vi "myRIO_BRig_RT_dataExp_laser1_Power_max.vi"() -> (2 "output_laser1_Power_max":i32)   [LabVIEW 2014]
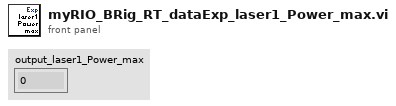
[diagram p1: front panel]
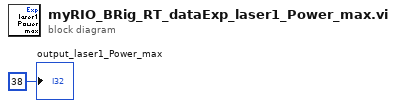
[diagram p0: block diagram]
diagram:
  "output_laser1_Power_max" <- 38 ("output_iBlock")
